vi "VINameProperty.vi"(11 "VIIn":refnum<vi>) -> (2 "Name":string, 3 "VIOut":refnum<vi>)   [LabVIEW 2021, in "YActor.lvclass"]
uses:
  YActor.lvclass
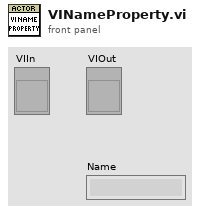
[diagram p1: front panel]
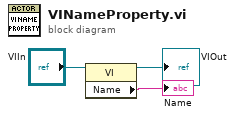
[diagram p0: block diagram]
diagram:
  n1 = property class="VI"(reference="VIIn") -> (reference out=→"VIOut":refnum<vi>, "Name"=→"Name":string)  [unwired: 1 in, 1 out]
